vi "Main Tclk.vi"() -> ()   [LabVIEW 2018] (continued)
            n5536 = call "2D array edit.vi"("Auto close (s)"=u32 15, "Display Format:Precision"=u8 3, "Rows"=w5117, "Columns"=w5118, "Caption.Text"="Focus Index", "Input array"=w5115) -> ()  [unwired: 5 in, 1 out]
          }
          event "Pre-reheat Y stig": Mouse Down {
            n5537 = event-data() -> ()  [unwired: 9 out]
            n5538 = local read "Pre-reheat Y stig"() -> (w5122:sgl[][])
            n5539 = local read "SEM Scan Parameters"() -> (w5126:T26)
            n5540 = Unbundle By Name(w5126) -> ("X tiles"=w5125:u8, "Y tiles"=w5124:u8)
            n5541 = call "2D array edit.vi"("Auto close (s)"=u32 15, "Display Format:Precision"=u8 2, "Rows"=w5124, "Columns"=w5125, "Caption.Text"="Pre-reheat Y stig (%)", "Input array"=w5122) -> ()  [unwired: 5 in, 1 out]
          }
          event "Align failed array": Mouse Down {
            n5542 = event-data() -> ()  [unwired: 9 out]
            n5543 = local read "Align failed array"() -> (w5129:bool[][])
            n5544 = call "2D boolean array show.vi"("Input array"=w5129, "Caption.Text"="Align failed", "Colors [4]"=cluster{u32, u32}[] [{5898240, 5898240}, {16711680, 16711680}, {1985280, 1985280}, {6618880, 6618880}] ("Colors [4] 3")) -> ()  [unwired: 8 in]
          }
          event "AF Success tiled": Mouse Down {
            n5545 = event-data() -> ()  [unwired: 9 out]
            n5546 = local read "AF Success tiled"() -> (w5132:bool[][])
            n5547 = call "2D boolean array show.vi"("Input array"=w5132, "Caption.Text"="Auto Focus Success", "Colors [4]"=cluster{u32, u32}[] [{1985280, 1985280}, {6618880, 6618880}, {1985280, 1985280}, {6618880, 6618880}]) -> ()  [unwired: 8 in]
          }
          event "ASX Success tiled": Mouse Down {
            n5548 = event-data() -> ()  [unwired: 9 out]
            n5549 = local read "ASX Success tiled"() -> (w5135:bool[][])
            n5550 = call "2D boolean array show.vi"("Input array"=w5135, "Caption.Text"="Auto Stig X Success", "Colors [4]"=cluster{u32, u32}[] [{1985280, 1985280}, {6618880, 6618880}, {1985280, 1985280}, {6618880, 6618880}]) -> ()  [unwired: 8 in]
          }
          event "ASY Success tiled": Mouse Down {
            n5551 = event-data() -> ()  [unwired: 9 out]
            n5552 = local read "ASY Success tiled"() -> (w5138:bool[][])
            n5553 = call "2D boolean array show.vi"("Input array"=w5138, "Caption.Text"="Auto Stig Y Success", "Colors [4]"=cluster{u32, u32}[] [{1985280, 1985280}, {6618880, 6618880}, {1985280, 1985280}, {6618880, 6618880}]) -> ()  [unwired: 8 in]
          }
          event "AAX Success tiled": Mouse Down {
            n5554 = event-data() -> ()  [unwired: 9 out]
            n5555 = local read "AAX Success tiled"() -> (w5141:bool[][])
            n5556 = call "2D boolean array show.vi"("Input array"=w5141, "Caption.Text"="Auto Align X Success", "Colors [4]"=cluster{u32, u32}[] [{1985280, 1985280}, {6618880, 6618880}, {1985280, 1985280}, {6618880, 6618880}]) -> ()  [unwired: 8 in]
          }
          event "AAY Success tiled": Mouse Down {
            n5557 = event-data() -> ()  [unwired: 9 out]
            n5558 = local read "AAY Success tiled"() -> (w5144:bool[][])
            n5559 = call "2D boolean array show.vi"("Input array"=w5144, "Caption.Text"="Auto Align Y Success", "Colors [4]"=cluster{u32, u32}[] [{1985280, 1985280}, {6618880, 6618880}, {1985280, 1985280}, {6618880, 6618880}]) -> ()  [unwired: 8 in]
          }
          event "Best WD (mm) tiled": Mouse Down {
            n5560 = event-data() -> ()  [unwired: 9 out]
            n5561 = local read "Best WD (mm) tiled"() -> (w5147:dbl[][])
            n5562 = local read "SEM Scan Parameters"() -> (w5151:T26)
            n5563 = Unbundle By Name(w5151) -> ("X tiles"=w5150:u8, "Y tiles"=w5149:u8)
            n5564 = call "2D array edit.vi"("Auto close (s)"=u32 15, "Display Format:Precision"=u8 4, "Rows"=w5149, "Columns"=w5150, "Caption.Text"="Best WD (mm)", "Input array"=w5147) -> ()  [unwired: 5 in, 1 out]
          }
          event "Best Stig X (%) tiled": Mouse Down {
            n5565 = event-data() -> ()  [unwired: 9 out]
            n5566 = local read "Best Stig X (%) tiled"() -> (w5154:dbl[][])
            n5567 = local read "SEM Scan Parameters"() -> (w5158:T26)
            n5568 = Unbundle By Name(w5158) -> ("X tiles"=w5157:u8, "Y tiles"=w5156:u8)
            n5569 = call "2D array edit.vi"("Auto close (s)"=u32 15, "Display Format:Precision"=u8 2, "Rows"=w5156, "Columns"=w5157, "Caption.Text"="Best Stig X (%)", "Input array"=w5154) -> ()  [unwired: 5 in, 1 out]
          }
          event "Best Stig Y (%) tiled": Mouse Down {
            n5570 = event-data() -> ()  [unwired: 9 out]
            n5571 = local read "Best Stig Y (%) tiled"() -> (w5161:dbl[][])
            n5572 = local read "SEM Scan Parameters"() -> (w5165:T26)
            n5573 = Unbundle By Name(w5165) -> ("X tiles"=w5164:u8, "Y tiles"=w5163:u8)
            n5574 = call "2D array edit.vi"("Auto close (s)"=u32 15, "Display Format:Precision"=u8 2, "Rows"=w5163, "Columns"=w5164, "Caption.Text"="Best Stig Y (%)", "Input array"=w5161) -> ()  [unwired: 5 in, 1 out]
          }
          event "Best Aln X (%) tiled": Mouse Down {
            n5575 = event-data() -> ()  [unwired: 9 out]
            n5576 = local read "Best Aln X (%) tiled"() -> (w5168:dbl[][])
            n5577 = local read "SEM Scan Parameters"() -> (w5172:T26)
            n5578 = Unbundle By Name(w5172) -> ("X tiles"=w5171:u8, "Y tiles"=w5170:u8)
            n5579 = call "2D array edit.vi"("Auto close (s)"=u32 15, "Display Format:Precision"=u8 2, "Rows"=w5170, "Columns"=w5171, "Caption.Text"="Best Align X (%)", "Input array"=w5168) -> ()  [unwired: 5 in, 1 out]
          }
          event "Best Aln Y (%) tiled": Mouse Down {
            n5580 = event-data() -> ()  [unwired: 9 out]
            n5581 = local read "Best Aln Y (%) tiled"() -> (w5175:dbl[][])
            n5582 = local read "SEM Scan Parameters"() -> (w5179:T26)
            n5583 = Unbundle By Name(w5179) -> ("X tiles"=w5178:u8, "Y tiles"=w5177:u8)
            n5584 = call "2D array edit.vi"("Auto close (s)"=u32 15, "Display Format:Precision"=u8 2, "Rows"=w5177, "Columns"=w5178, "Caption.Text"="Best Align Y (%)", "Input array"=w5175) -> ()  [unwired: 5 in, 1 out]
          }
          event "Auto Focus Graph": Mouse Down {
            n5585 = event-data() -> ("PlatMods"=w5191:T77)  [unwired: 8 out]
            n5586 = Unbundle By Name(w5191) -> ("Shift"=w5190:bool)
            n5587 = local read "AF Graph scales tiled"() -> (w5187:cluster{sgl, sgl, sgl, sgl}[][])
            n5588 = local read "Auto Focus Graph tiled"() -> (w5196:T4)
            n5589 = local read "AF Y tile"() -> (w5195:u8)
            n5590 = local read "AF X tile"() -> (w5194:u8)
            n5591 = local read "SEM Scan Parameters"() -> (w5193:T26)
            n5592 = Unbundle By Name(w5193) -> ("X tiles"=w5192:u8, "Y tiles"=w5189:u8)
            n5593 = case shown="True" w5190 {
              tunnel: w5196 -> [w5206 w5215]
              tunnel: w5195 -> [w5199 w5213]
              tunnel: w5194 -> [w5205 w5208]
              tunnel: w5192 -> [w5203 _]
              tunnel: w5189 -> [_ w5214]
              tunnel: [w5202 w5212] -> w5188
              tunnel: w5187 -> [w5201 w5211]
              tunnel: [w5200 w5210] -> w5186
              tunnel: [w5197 w5207] -> w5181
              frame False {
                n5594 = Increment(x=w5205) -> (x+1=w5204:u8)
                n5595 = Quotient & Remainder(x=w5204, y=w5203) -> (x-y*floor(x/y)=w5198:u8)  [unwired: 1 out]
                n5596 = Index Array(array=w5201, index (row)=w5199, index (col)=w5198) -> (element=w5200:cluster{sgl, sgl, sgl, sgl})
                n5597 = Index Array(array=w5206, index (dim 0)=w5199, index (dim 1)=w5198) -> (element=w5202:T76)  [unwired: 1 in]
                n5598 = local write "AF X tile"(w5198) -> ()
                n5599 = Build Array(w5199, w5198) -> (w5197:u8[])
              }
              frame True {
                n5600 = Increment(x=w5213) -> (x+1=w5216:u8)
                n5601 = Quotient & Remainder(x=w5216, y=w5214) -> (x-y*floor(x/y)=w5209:u8)  [unwired: 1 out]
                n5602 = Index Array(array=w5211, index (row)=w5209, index (col)=w5208) -> (element=w5210:cluster{sgl, sgl, sgl, sgl})
                n5603 = Index Array(array=w5215, index (dim 0)=w5209, index (dim 1)=w5208) -> (element=w5212:T76)  [unwired: 1 in]
                n5604 = local write "AF Y tile"(w5209) -> ()
                n5605 = Build Array(w5209, w5208) -> (w5207:u8[])
              }
            }
            n5606 = Unbundle(w5186) -> (w5185:sgl, w5184:sgl, w5183:sgl, w5182:sgl)
            n5607 = local write "Auto Focus Graph"(w5188) -> ()
            n5608 = property on="AF Success tiled" class="Arr (strict)"("Index Values"=w5181) -> ()  [unwired: 2 in, 2 out]
            n5609 = property on="Best WD (mm) tiled" class="Arr (strict)"("Index Values"=w5181) -> ()  [unwired: 2 in, 2 out]
            n5610 = property on="Best WD FI tiled" class="Arr (strict)"("Index Values"=w5181) -> ()  [unwired: 2 in, 2 out]
            n5611 = property on="Auto Focus Graph" class="XYGraph (strict)"("XScale.Maximum"=w5185, "XScale.Minimum"=w5184, "YScale.Maximum"=w5183, "YScale.Minimum"=w5182) -> ()  [unwired: 2 in, 2 out]
          }
          event "Auto Stig X": Mouse Down {
            n5612 = event-data() -> ("PlatMods"=w5227:T77)  [unwired: 8 out]
            n5613 = Unbundle By Name(w5227) -> ("Shift"=w5226:bool)
            n5614 = local read "ASX Graph scales tiled"() -> (w5223:cluster{sgl, sgl, sgl, sgl}[][])
            n5615 = local read "ASX Graph tiled"() -> (w5232:T4)
            n5616 = local read "ASX Y tile"() -> (w5231:u8)
            n5617 = local read "ASX X tile"() -> (w5230:u8)
            n5618 = local read "SEM Scan Parameters"() -> (w5229:T26)
            n5619 = Unbundle By Name(w5229) -> ("X tiles"=w5228:u8, "Y tiles"=w5225:u8)
            n5620 = case shown="False" w5226 {
              tunnel: w5232 -> [w5242 w5251]
              tunnel: w5231 -> [w5235 w5249]
              tunnel: w5230 -> [w5241 w5244]
              tunnel: w5228 -> [w5239 _]
              tunnel: w5225 -> [_ w5250]
              tunnel: [w5238 w5248] -> w5224
              tunnel: w5223 -> [w5237 w5247]
              tunnel: [w5236 w5246] -> w5222
              tunnel: [w5233 w5243] -> w5217
              frame False {
                n5621 = Increment(x=w5241) -> (x+1=w5240:u8)
                n5622 = Quotient & Remainder(x=w5240, y=w5239) -> (x-y*floor(x/y)=w5234:u8)  [unwired: 1 out]
                n5623 = Index Array(array=w5237, index (row)=w5235, index (col)=w5234) -> (element=w5236:cluster{sgl, sgl, sgl, sgl})
                n5624 = Index Array(array=w5242, index (dim 0)=w5235, index (dim 1)=w5234) -> (element=w5238:T76)  [unwired: 1 in]
                n5625 = local write "ASX X tile"(w5234) -> ()
                n5626 = Build Array(w5235, w5234) -> (w5233:u8[])
              }
              frame True {
                n5627 = Increment(x=w5249) -> (x+1=w5252:u8)
                n5628 = Quotient & Remainder(x=w5252, y=w5250) -> (x-y*floor(x/y)=w5245:u8)  [unwired: 1 out]
                n5629 = Index Array(array=w5247, index (row)=w5245, index (col)=w5244) -> (element=w5246:cluster{sgl, sgl, sgl, sgl})
                n5630 = Index Array(array=w5251, index (dim 0)=w5245, index (dim 1)=w5244) -> (element=w5248:T76)  [unwired: 1 in]
                n5631 = local write "ASX Y tile"(w5245) -> ()
                n5632 = Build Array(w5245, w5244) -> (w5243:u8[])
              }
            }
            n5633 = Unbundle(w5222) -> (w5221:sgl, w5220:sgl, w5219:sgl, w5218:sgl)
            n5634 = local write "Auto Stig X"(w5224) -> ()
            n5635 = property on="ASX Success tiled" class="Arr (strict)"("Index Values"=w5217) -> ()  [unwired: 2 in, 2 out]
            n5636 = property on="Best Stig X (%) tiled" class="Arr (strict)"("Index Values"=w5217) -> ()  [unwired: 2 in, 2 out]
            n5637 = property on="Best Stig X FI tiled" class="Arr (strict)"("Index Values"=w5217) -> ()  [unwired: 2 in, 2 out]
            n5638 = property on="Auto Stig X" class="XYGraph (strict)"("XScale.Maximum"=w5221, "XScale.Minimum"=w5220, "YScale.Maximum"=w5219, "YScale.Minimum"=w5218) -> ()  [unwired: 2 in, 2 out]
          }
          event "Auto Stig Y": Mouse Down {
            n5639 = event-data() -> ("PlatMods"=w5263:T77)  [unwired: 8 out]
            n5640 = Unbundle By Name(w5263) -> ("Shift"=w5262:bool)
            n5641 = local read "ASY Graph scales tiled"() -> (w5259:cluster{sgl, sgl, sgl, sgl}[][])
            n5642 = local read "ASY Graph tiled"() -> (w5268:T4)
            n5643 = local read "ASY Y tile"() -> (w5267:u8)
            n5644 = local read "ASY X tile"() -> (w5266:u8)
            n5645 = local read "SEM Scan Parameters"() -> (w5265:T26)
            n5646 = Unbundle By Name(w5265) -> ("X tiles"=w5264:u8, "Y tiles"=w5261:u8)
            n5647 = case shown="True" w5262 {
              tunnel: w5268 -> [w5278 w5287]
              tunnel: w5267 -> [w5271 w5285]
              tunnel: w5266 -> [w5277 w5280]
              tunnel: w5264 -> [w5275 _]
              tunnel: w5261 -> [_ w5286]
              tunnel: [w5274 w5284] -> w5260
              tunnel: w5259 -> [w5273 w5283]
              tunnel: [w5272 w5282] -> w5258
              tunnel: [w5269 w5279] -> w5253
              frame False {
                n5648 = Increment(x=w5277) -> (x+1=w5276:u8)
                n5649 = Quotient & Remainder(x=w5276, y=w5275) -> (x-y*floor(x/y)=w5270:u8)  [unwired: 1 out]
                n5650 = Index Array(array=w5273, index (row)=w5271, index (col)=w5270) -> (element=w5272:cluster{sgl, sgl, sgl, sgl})
                n5651 = Index Array(array=w5278, index (dim 0)=w5271, index (dim 1)=w5270) -> (element=w5274:T76)  [unwired: 1 in]
                n5652 = local write "ASY X tile"(w5270) -> ()
                n5653 = Build Array(w5271, w5270) -> (w5269:u8[])
              }
              frame True {
                n5654 = Increment(x=w5285) -> (x+1=w5288:u8)
                n5655 = Quotient & Remainder(x=w5288, y=w5286) -> (x-y*floor(x/y)=w5281:u8)  [unwired: 1 out]
                n5656 = Index Array(array=w5283, index (row)=w5281, index (col)=w5280) -> (element=w5282:cluster{sgl, sgl, sgl, sgl})
                n5657 = Index Array(array=w5287, index (dim 0)=w5281, index (dim 1)=w5280) -> (element=w5284:T76)  [unwired: 1 in]
                n5658 = local write "ASY Y tile"(w5281) -> ()
                n5659 = Build Array(w5281, w5280) -> (w5279:u8[])
              }
            }
            n5660 = Unbundle(w5258) -> (w5257:sgl, w5256:sgl, w5255:sgl, w5254:sgl)
            n5661 = local write "Auto Stig Y"(w5260) -> ()
            n5662 = property on="ASY Success tiled" class="Arr (strict)"("Index Values"=w5253) -> ()  [unwired: 2 in, 2 out]
            n5663 = property on="Best Stig Y (%) tiled" class="Arr (strict)"("Index Values"=w5253) -> ()  [unwired: 2 in, 2 out]
            n5664 = property on="Best Stig Y FI tiled" class="Arr (strict)"("Index Values"=w5253) -> ()  [unwired: 2 in, 2 out]
            n5665 = property on="Auto Stig Y" class="XYGraph (strict)"("XScale.Maximum"=w5257, "XScale.Minimum"=w5256, "YScale.Maximum"=w5255, "YScale.Minimum"=w5254) -> ()  [unwired: 2 in, 2 out]
          }
          event "Auto Aln X": Mouse Down {
            n5666 = event-data() -> ("PlatMods"=w5299:T77)  [unwired: 8 out]
            n5667 = Unbundle By Name(w5299) -> ("Shift"=w5298:bool)
            n5668 = local read "AAX Graph scales tiled"() -> (w5295:cluster{sgl, sgl, sgl, sgl}[][])
            n5669 = local read "AAX Graph tiled"() -> (w5304:T4)
            n5670 = local read "AAX Y tile"() -> (w5303:u8)
            n5671 = local read "AAX X tile"() -> (w5302:u8)
            n5672 = local read "SEM Scan Parameters"() -> (w5301:T26)
            n5673 = Unbundle By Name(w5301) -> ("X tiles"=w5300:u8, "Y tiles"=w5297:u8)
            n5674 = case shown="False" w5298 {
              tunnel: w5304 -> [w5314 w5323]
              tunnel: w5303 -> [w5307 w5321]
              tunnel: w5302 -> [w5313 w5316]
              tunnel: w5300 -> [w5311 _]
              tunnel: w5297 -> [_ w5322]
              tunnel: [w5310 w5320] -> w5296
              tunnel: w5295 -> [w5309 w5319]
              tunnel: [w5308 w5318] -> w5294
              tunnel: [w5305 w5315] -> w5289
              frame False {
                n5675 = Increment(x=w5313) -> (x+1=w5312:u8)
                n5676 = Quotient & Remainder(x=w5312, y=w5311) -> (x-y*floor(x/y)=w5306:u8)  [unwired: 1 out]
                n5677 = local write "AAX X tile"(w5306) -> ()
                n5678 = Index Array(array=w5309, index (row)=w5307, index (col)=w5306) -> (element=w5308:cluster{sgl, sgl, sgl, sgl})
                n5679 = Index Array(array=w5314, index (dim 0)=w5307, index (dim 1)=w5306) -> (element=w5310:T76)  [unwired: 1 in]
                n5680 = Build Array(w5307, w5306) -> (w5305:u8[])
              }
              frame True {
                n5681 = Increment(x=w5321) -> (x+1=w5324:u8)
                n5682 = Quotient & Remainder(x=w5324, y=w5322) -> (x-y*floor(x/y)=w5317:u8)  [unwired: 1 out]
                n5683 = local write "AAX Y tile"(w5317) -> ()
                n5684 = Index Array(array=w5319, index (row)=w5317, index (col)=w5316) -> (element=w5318:cluster{sgl, sgl, sgl, sgl})
                n5685 = Index Array(array=w5323, index (dim 0)=w5317, index (dim 1)=w5316) -> (element=w5320:T76)  [unwired: 1 in]
                n5686 = Build Array(w5317, w5316) -> (w5315:u8[])
              }
            }
            n5687 = Unbundle(w5294) -> (w5293:sgl, w5292:sgl, w5291:sgl, w5290:sgl)
            n5688 = property on="AAX Success tiled" class="Arr (strict)"("Index Values"=w5289) -> ()  [unwired: 2 in, 2 out]
            n5689 = property on="Best Aln X (%) tiled" class="Arr (strict)"("Index Values"=w5289) -> ()  [unwired: 2 in, 2 out]
            n5690 = property on="Best Aln X FI tiled" class="Arr (strict)"("Index Values"=w5289) -> ()  [unwired: 2 in, 2 out]
            n5691 = local write "Auto Aln X"(w5296) -> ()
            n5692 = property on="Auto Aln X" class="XYGraph (strict)"("XScale.Maximum"=w5293, "XScale.Minimum"=w5292, "YScale.Maximum"=w5291, "YScale.Minimum"=w5290) -> ()  [unwired: 2 in, 2 out]
          }
          event "Auto Aln Y": Mouse Down {
            n5693 = event-data() -> ("PlatMods"=w5335:T77)  [unwired: 8 out]
            n5694 = Unbundle By Name(w5335) -> ("Shift"=w5334:bool)
            n5695 = local read "AAY Graph scales tiled"() -> (w5331:cluster{sgl, sgl, sgl, sgl}[][])
            n5696 = local read "AAY Graph tiled"() -> (w5340:T4)
            n5697 = local read "AAY Y tile"() -> (w5339:u8)
            n5698 = local read "AAY X tile"() -> (w5338:u8)
            n5699 = local read "SEM Scan Parameters"() -> (w5337:T26)
            n5700 = Unbundle By Name(w5337) -> ("X tiles"=w5336:u8, "Y tiles"=w5333:u8)
            n5701 = case shown="True" w5334 {
              tunnel: w5340 -> [w5350 w5359]
              tunnel: w5339 -> [w5343 w5357]
              tunnel: w5338 -> [w5349 w5352]
              tunnel: w5336 -> [w5347 _]
              tunnel: w5333 -> [_ w5358]
              tunnel: [w5346 w5356] -> w5332
              tunnel: w5331 -> [w5345 w5355]
              tunnel: [w5344 w5354] -> w5330
              tunnel: [w5341 w5351] -> w5325
              frame False {
                n5702 = Increment(x=w5349) -> (x+1=w5348:u8)
                n5703 = Quotient & Remainder(x=w5348, y=w5347) -> (x-y*floor(x/y)=w5342:u8)  [unwired: 1 out]
                n5704 = local write "AAY X tile"(w5342) -> ()
                n5705 = Index Array(array=w5345, index (row)=w5343, index (col)=w5342) -> (element=w5344:cluster{sgl, sgl, sgl, sgl})
                n5706 = Index Array(array=w5350, index (dim 0)=w5343, index (dim 1)=w5342) -> (element=w5346:T76)  [unwired: 1 in]
                n5707 = Build Array(w5343, w5342) -> (w5341:u8[])
              }
              frame True {
                n5708 = Increment(x=w5357) -> (x+1=w5360:u8)
                n5709 = Quotient & Remainder(x=w5360, y=w5358) -> (x-y*floor(x/y)=w5353:u8)  [unwired: 1 out]
                n5710 = local write "AAY Y tile"(w5353) -> ()
                n5711 = Index Array(array=w5355, index (row)=w5353, index (col)=w5352) -> (element=w5354:cluster{sgl, sgl, sgl, sgl})
                n5712 = Index Array(array=w5359, index (dim 0)=w5353, index (dim 1)=w5352) -> (element=w5356:T76)  [unwired: 1 in]
                n5713 = Build Array(w5353, w5352) -> (w5351:u8[])
              }
            }
            n5714 = Unbundle(w5330) -> (w5329:sgl, w5328:sgl, w5327:sgl, w5326:sgl)
            n5715 = property on="AAY Success tiled" class="Arr (strict)"("Index Values"=w5325) -> ()  [unwired: 2 in, 2 out]
            n5716 = property on="Best Aln Y (%) tiled" class="Arr (strict)"("Index Values"=w5325) -> ()  [unwired: 2 in, 2 out]
            n5717 = property on="Best Aln Y FI tiled" class="Arr (strict)"("Index Values"=w5325) -> ()  [unwired: 2 in, 2 out]
            n5718 = local write "Auto Aln Y"(w5332) -> ()
            n5719 = property on="Auto Aln Y" class="XYGraph (strict)"("XScale.Maximum"=w5329, "XScale.Minimum"=w5328, "YScale.Maximum"=w5327, "YScale.Minimum"=w5326) -> ()  [unwired: 2 in, 2 out]
          }
        }
        n5720 = Unbundle By Name(w2953) -> ("status"=w2951:bool)
        n5721 = Or(x=w2951, y=w2950) -> (x .or. y?=w2952:bool)
      }
      n5722 = while {
        stop <- w768 stop-if-true
        n5723 = Wait Until Next ms Multiple(millisecond multiple=u32 100) -> ()  [unwired: 1 out]
        n5724 = case shown="True" "Start Reheat" {
          frame False {
          }
          frame True {
            n5725 = stacked-sequence {
              frame #0 {
                n5726 = local read "Milling para"() -> (w773:T35)
                n5727 = local read "Auto reheat running"() -> (w771:bool)
                n5728 = Unbundle By Name(w773) -> ("Auto Profile"=w772:bool)
                n5729 = And(x=w772, y=w771) -> (x .and. y?=w770:bool)
                n5730 = case shown="True" w770 {
                  frame False {
                  }
                  frame True {
                    n5731 = stacked-sequence {
                      frame #0 {
                        n5732 = local read "Post #1up"() -> (w778:tag)
                        n5733 = local read "Post #1down"() -> (w777:tag)
                        n5734 = local read "Post #2up"() -> (w776:tag)
                        n5735 = local read "Post #2down"() -> (w775:tag)
                        n5736 = local write "FIB Profile"(TRUE ("FIB Profile")) -> ()
                        n5737 = local write "Enable logging"(FALSE ("Enable logging")) -> ()
                        n5738 = call "SEM shutter.vi"("Shutter close"=TRUE, "Shutter AO4"=w775, "Shutter AO3"=w776, "Shutter AO2"=w777, "Shutter AO1"=w778) -> ()  [unwired: 6 in, 1 out]
                      }
                      frame #1 {
                        n5739 = Wait (ms)(milliseconds to wait=u32 10000) -> ()  [unwired: 1 out]
                      }
                      frame #2 {
                        n5740 = local read "Machine Type"() -> (w782:u8)
                        n5741 = case shown="0, Default" w782 {
                          frame 0, Default {
                            w783 = sgl 90.0 ("UL-Ang")
                            n5742 = local read "HV Data Output"() -> (w799:T18)
                            n5743 = local read "Active logging channels"() -> (w787:string)
                            n5744 = local read "FIB HW Config"() -> (w790:T23)
                            n5745 = local read "FIB Options"() -> (w789:T33)
                            n5746 = local read "Milling para"() -> (w793:T35)
                            n5747 = local read "FIB profile X center (um)"() -> (w798:dbl)
                            n5748 = local read "FIB profile Y center (um)"() -> (w797:dbl)
                            n5749 = local read "FIB Scan Parameters"() -> (w792:T32)
                            n5750 = local read "Parameter Names"() -> (w786:string[])
                            n5751 = Bundle By Name(cluster=w792, "Frame line rampdown ratio"=0.0, "Oversampling"=u16 5) -> (w788:T32)
                            n5752 = Bundle By Name(cluster=w793, "X size (um)"=sgl 0.1, "Z size (um)"=sgl 10.0 ("Y size (um)"), "X center (um)"=w798, "Z center (um)"=w797, "UL-Ang"=w783, "UR-Ang"=w783) -> (w794:T35)
                            n5753 = call "FIB profile.vi"("HV Data Output"=w799, "Parameter Names"=w786, "Active logging channels"=w787, "Scan Para"=w788, "Milling para"=w794, "Options"=w789, "HW Config"=w790) -> ("Measurements"=w785:dbl[][])  [unwired: 2 in, 2 out]
                            n5754 = local write "Measurements"(w785) -> ()
                          }
                          frame 2 {
                            w800 = sgl 90.0 ("UL-Ang")
                            n5755 = local read "Active logging channels"() -> (w805:string)
                            n5756 = local read "FIB HW Config"() -> (w808:T23)
                            n5757 = local read "FIB Options"() -> (w807:T33)
                            n5758 = local read "Milling para"() -> (w811:T35)
                            n5759 = local read "FIB profile X center (um)"() -> (w816:dbl)
                            n5760 = local read "FIB profile Y center (um)"() -> (w815:dbl)
                            n5761 = local read "FIB Scan Parameters"() -> (w810:T32)
                            n5762 = local read "Parameter Names"() -> (w804:string[])
                            n5763 = local read "Capella HV Data Output"() -> (w801:T17)
                            n5764 = Bundle By Name(cluster=w810, "Frame line rampdown ratio"=0.0, "Oversampling"=u16 5) -> (w806:T32)
                            n5765 = Bundle By Name(cluster=w811, "X size (um)"=sgl 0.1, "Z size (um)"=sgl 10.0 ("Y size (um)"), "X center (um)"=w816, "Z center (um)"=w815, "UL-Ang"=w800, "UR-Ang"=w800) -> (w812:T35)
                            n5766 = call "FIB profile.vi"("Capella HV Data Output"=w801, "Parameter Names"=w804, "Active logging channels"=w805, "Scan Para"=w806, "Milling para"=w812, "Options"=w807, "HW Config"=w808) -> ("Measurements"=w803:dbl[][])  [unwired: 2 in, 2 out]
                            n5767 = local write "Measurements"(w803) -> ()
                          }
                        }
                      }
                      frame #3 {
                        n5768 = local write "FIB Profile"(FALSE ("FIB Profile")) -> ()
                        n5769 = local write "Enable logging"(TRUE ("Enable logging")) -> ()
                      }
                    }
                  }
                }
              }
              frame #1 {
                n5770 = local read "Machine Type"() -> (w819:u8)
                n5771 = case shown="2" w819 {
                  selector: w819 -> [w820 _ w911]
                  frame 0, Default {
                    n5772 = stacked-sequence {
                      tunnel: w820 -> [_ _ _ _ _ _ _ _ w905]
                      frame #0 {
                        n5773 = local read "Reheat start file"() -> (w821:path)
                        n5774 = File/Directory Info(path=w821) -> (path out=w824:path, error out=w822:errorcluster)  [unwired: 1 in, 5 out]
                        n5775 = Unbundle By Name(w822) -> ("status"=w823:bool)
                        n5776 = case shown="False" w823 {
                          tunnel: w824 -> [w825 _]
                          frame False {
                            n5777 = Delete(path (use dialog)=w825) -> ()  [unwired: 4 in, 3 out]
                          }
                          frame True {
                          }
                        }
                      }
                      frame #1 {
                        n5778 = local read "Reheat complete file"() -> (w828:path)
                        n5779 = local read "Reheat stopped file"() -> (w827:path)
                        n5780 = local write "Reheat completed"(FALSE ("Reheat completed")) -> ()
                        n5781 = local write "Status Tabs"(T11."FIB" ("Status Tabs")) -> ()
                        n5782 = File/Directory Info(path=w828) -> (path out=w834:path, last mod=w830:timestamp, error out=w836:errorcluster)  [unwired: 1 in, 4 out]
                        n5783 = File/Directory Info(path=w827) -> (path out=w833:path, error out=w831:errorcluster)  [unwired: 1 in, 5 out]
                        n5784 = Unbundle By Name(w836) -> ("status"=w835:bool)
                        n5785 = Unbundle By Name(w831) -> ("status"=w832:bool)
                        n5786 = case shown="False" w835 {
                          tunnel: w834 -> [w839 _]
                          tunnel: w830 -> [w838 _]
                          frame False {
                            n5787 = Delete(path (use dialog)=w839) -> ()  [unwired: 4 in, 3 out]
                            "Last auto reheat" <- w838
                          }
                          frame True {
                          }
                        }
                        n5788 = case shown="False" w832 {
                          tunnel: w833 -> [w837 _]
                          frame False {
                            n5789 = Delete(path (use dialog)=w837) -> ()  [unwired: 4 in, 3 out]
                          }
                          frame True {
                          }
                        }
                      }
                      frame #2 {
                        n5790 = local read "Auto reheat running"() -> (w847:bool)
                        n5791 = Get Date/Time In Seconds() -> (seconds since 1Jan1904=w844:timestamp)
                        "Reheat time" <- w844
                        n5792 = local read "Last auto reheat"() -> (w843:timestamp)
                        n5793 = local read "Turn FIB Gun on"() -> (w840:bool)
                        n5794 = property on="Request to stop reheat" class="Bool (strict)"("DisabledEnum"=T44."Enabled" ("Disabled")) -> ()  [unwired: 2 in, 2 out]
                        n5795 = Subtract(x=w844, y=w843) -> (x-y=w851:dbl)
                        n5796 = expression code="x/60"(w851) -> (w850:dbl)
                        n5797 = Less Or Equal?(x=w850, y=120.0) -> (x <= y?=w848:bool)
                        n5798 = And(x=w847, y=w848) -> (x .and. y?=w842:bool)
                        n5799 = Or(x=w842, y=w840) -> (x .or. y?=w841:bool)
                        n5800 = case shown="True" w841 {
                          tunnel: "Reheat Parameters" -> [w853 w859]
                          tunnel: [w853 w855] -> w845
                          frame False {
                          }
                          frame True {
                            n5801 = Bundle By Name(cluster=w859, "Filament I (A)"=sgl 0.1, "Reheat time (s)"=sgl 1.0, "Calculate V/I slope"=FALSE, "Disable Reheat Retries"=TRUE) -> (w855:T1)
                          }
                        }
                        "Actual Reheat Parameters" <- w845
                      }
                      frame #3 {
                        n5802 = local read "Actual Reheat Parameters"() -> (w861:T1)
                        n5803 = call "Write FIB reheat file.vi"("Reheat Parameters"=w861) -> ()  [unwired: 11 in]
                        "Send reheat start email" <- TRUE
                      }
                      frame #4 {
                        n5804 = while {
                          stop <- w877 stop-if-true
                          n5805 = local read "Reheat complete file"() -> (w873:path)
                          n5806 = local read "Reheat stopped file"() -> (w874:path)
                          n5807 = Wait Until Next ms Multiple(millisecond multiple=u32 100) -> ()  [unwired: 1 out]
                          n5808 = File/Directory Info(path=w873) -> (path out=w869:path, error out=w868:errorcluster)  [unwired: 1 in, 5 out]
                          n5809 = File/Directory Info(path=w874) -> (path out=w870:path, error out=w871:errorcluster)  [unwired: 1 in, 5 out]
                          n5810 = local read "Stop"() -> (w878:bool)
                          n5811 = Unbundle By Name(w868) -> ("status"=w867:bool)
                          n5812 = Unbundle By Name(w871) -> ("status"=w872:bool)
                          n5813 = Not(x=w867) -> (.not. x?=w875:bool)
                          n5814 = Not(x=w872) -> (.not. x?=w876:bool)
                          n5815 = case shown="True" w875 {
                            selector: w875 -> [w885 w886]
                            tunnel: w869 -> [_ w887]
                            tunnel: [w885 w886] -> w864
                            frame False {
                            }
                            frame True {
                              "Reheat log file" <- w887
                            }
                          }
                          n5816 = case shown="True" w876 {
                            selector: w876 -> [w882 w883]
                            tunnel: w870 -> [_ w884]
                            tunnel: [w882 w883] -> w863
                            frame False {
                            }
                            frame True {
                              n5817 = local write "Reheat log file"(w884) -> ()
                            }
                          }
                          n5818 = Or(x=w864, y=w863) -> (x .or. y?=w866:bool)
                          n5819 = Or(x=w866, y=w878) -> (x .or. y?=w877:bool)
                          n5820 = case shown="True" "Stop Reheat" {
                            frame False {
                              n5821 = local write "Status message"("FIB reheat in progress..." ("Status message")) -> ()
                            }
                            frame True {
                              n5822 = local write "Status message"("Stopping FIB reheat" ("Status message")) -> ()
                              n5823 = call "Write FIB reheat file.vi"("Start"=FALSE) -> ()  [unwired: 11 in]
                            }
                          }
                        }
                      }
                      frame #5 {
                        n5824 = Wait (ms)(milliseconds to wait=u32 500) -> ()  [unwired: 1 out]
                      }
                      frame #6 {
                        w895 = u8 1 items=["HV Data", "Reheat"] ("Log file type")
                        n5825 = local read "Reheat log file"() -> (w897:path)
                        n5826 = call "Read FIB Log Files.vi"("Log file type"=w895, "Log file path"=w897) -> ("Reheat Output"=→"Reheat Output":T21)  [unwired: 8 in, 1 out]
                        n5827 = call "Read FIB Log Files.vi"("Log file path"=path "C:/Program Files (x86)/FEI Company/BDS/LogHVData.log") -> ("HV Data Output"=w890:T113)  [unwired: 9 in, 1 out]
                        n5828 = File/Directory Info(path=path "C:/Program Files (x86)/FEI Company/BDS/Reheat/Stop.txt" ("Log file path")) -> (path out=w894:path, error out=w892:errorcluster)  [unwired: 1 in, 5 out]
                        n5829 = local write "HV Data Output"(w890) -> ()
                        n5830 = Unbundle By Name(w892) -> ("status"=w893:bool)
                        n5831 = case shown="False" w893 {
                          tunnel: w894 -> [w898 _]
                          frame False {
                            n5832 = Delete(path (use dialog)=w898) -> ()  [unwired: 4 in, 3 out]
                          }
                          frame True {
                          }
                        }
                      }
                      frame #7 {
                        n5833 = local read "Stop Reheat"() -> (w901:bool)
                        n5834 = local read "Reheat Output"() -> (w900:T21)
                        n5835 = Unbundle By Name(w900) -> ("Reheat Success"=w899:bool)
                        n5836 = Select(t="Reheat Stopped" ("Status message"), s=w901, f="Reheat Completed" ("Status message")) -> (s? t:f=w904:string)
                        n5837 = local write "Status message"(w904) -> ()
                        n5838 = local write "Start FIB HV DataLog"(w899) -> ()
                      }
                      frame #8 {
                        n5839 = local read "Reheat Output"() -> (w908:T21)
                        n5840 = local read "FIB Reheat Log Files"() -> (w907:path)
                        n5841 = local read "Reheat time"() -> (w906:timestamp)
                        n5842 = local read "HV Data Output"() -> (w910:T18)
                        n5843 = local read "Actual Reheat Parameters"() -> (w909:T1)
                        n5844 = call "Write FIB reheat log.vi"("HV Data Output"=w910, "Reheat Output"=w908, "Reheat Parameters"=w909, "Reheat time"=w906, "Machine Type"=w905, "Log file path"=w907) -> ()  [unwired: 6 in]
                      }
                    }
                  }
                  frame 1 {
                  }
                  frame 2 {
                    n5845 = stacked-sequence {
                      tunnel: w911 -> [_ _ _ _ _ _ w1029]
                      frame #0 {
                        n5846 = local read "Api"() -> (w914:refnum<k7>)
                        n5847 = local write "Status Tabs"(T11."FIB" ("Status Tabs")) -> ()
                        n5848 = local write "Reheat completed"(FALSE ("Reheat completed")) -> ()
                        n5849 = property on="Request to stop reheat" class="Bool (strict)"("DisabledEnum"=T44."Enabled" ("Disabled")) -> ()  [unwired: 2 in, 2 out]
                        n5850 = call "SmartSEM Remote API set float.vi"("vValue"=sgl 1.0, "lpszParam"="DP_FIB_BLANKED", "Api"=w914) -> ("error out"=w912:errorcluster, "Api out"=w913:refnum<k7>)  [unwired: 7 in]
                        n5851 = call "SmartSEM Remote API get FIB HV data.vi"("error in"=w912, "Api in"=w913) -> ("Capella HV Data Output"=w917:T17)  [unwired: 6 in, 3 out]
                        n5852 = local write "Capella HV Data Output"(w917) -> ()
                      }
                      frame #1 {
                        n5853 = Get Date/Time In Seconds() -> (seconds since 1Jan1904=w921:timestamp)
                        n5854 = local read "Api"() -> (w924:refnum<k7>)
                        n5855 = local write "Send reheat start email"(TRUE) -> ()
                        n5856 = local write "Reheat time"(w921) -> ()
                        n5857 = invoke class="_EMApi" method="Execute"(reference=w924, "lpszCommand"="CMD_FIB_TC_MH_REQ_START") -> ()  [unwired: 2 in, 4 out]
                      }
                      frame #2 {
                        n5858 = Wait (ms)(milliseconds to wait=u32 30000) -> ()  [unwired: 1 out]
                        n5859 = local write "Status message"("FIB reheat in progress..." ("Status message")) -> ()
                      }
                      frame #3 {
                        n5860 = while {
                          stop <- w932 stop-if-true
                          n5861 = local read "Api"() -> (w929:refnum<k7>)
                          n5862 = call "SmartSEM Remote API FIB gun state.vi"("Api"=w929) -> ("FIB Gun State"=w931:string, "Api out"=w927:refnum<k7>)  [unwired: 8 in, 1 out]
                          n5863 = Wait Until Next ms Multiple(millisecond multiple=u32 100) -> ()  [unwired: 1 out]
                          n5864 = case shown="\"FIB Emissin Failed\"" w931 {
                            tunnel: [FALSE ("x") TRUE ("x") w949] -> w930
                            tunnel: w927 -> [_ _ w948]
                            frame "", Default {
                            }
                            frame "FIB Emissin Failed" {
                              n5865 = Get Date/Time In Seconds() -> (seconds since 1Jan1904=w938:timestamp)
                              n5866 = Get Date/Time String(seconds (now)=w938) -> (date string=w939:string, time string=w940:string)  [unwired: 2 in]
                              n5867 = Concatenate Strings(w939, " " ("string"), w940) -> (w937:string)
                              n5868 = local read "Reheat Output"() -> (w942:T21)
                              n5869 = Bundle By Name(cluster=w942, "Reheat finish time"=w937, "Reheat Success"=FALSE) -> (w943:T21)
                              n5870 = local write "Reheat Output"(w943) -> ()
                            }
                            frame "Regulating" {
                              n5871 = call "SmartSEM Remote API get string.vi"("lpszParam"="DP_FIB_PURGE_STATE", "Api"=w948) -> ("data"=w946:string, "Api out"=w945:refnum<k7>)  [unwired: 7 in, 1 out]
                              n5872 = case shown="\"Idle\"" w946 {
                                tunnel: w945 -> [_ w952]
                                tunnel: [FALSE ("x") w951] -> w949
                                frame "", Default {
                                }
                                frame "Idle" {
                                n5873 = stacked-sequence {
                                tunnel: w952 -> [w955 _ w960 _]
                                tunnel: [_ _ _ TRUE ("x")] -> w951
                                frame #0 {
                                n5874 = local read "FIB HW Config"() -> (w954:T23)
                                n5875 = Unbundle By Name(w954) -> ("Beam blank"=w953:tag)
                                n5876 = call "FIB beam blank.vi"("Api"=w955, "Beam blanked"=TRUE, "lines"=w953) -> ()  [unwired: 2 in, 1 out]
                                }
                                frame #1 {
                                n5877 = Wait (ms)(milliseconds to wait=u32 60000) -> ()  [unwired: 1 out]
                                n5878 = local write "Status message"("Stablizing for 1 min ..." ("Status message")) -> ()
                                }
                                frame #2 {
                                n5879 = call "SmartSEM Remote API FIB VI slope.vi"("Api"=w960) -> ("V/I slope"=w961:sgl)  [unwired: 8 in, 2 out]
                                n5880 = local write "Status message"("Measuring FIB V/I slope ..." ("Status message")) -> ()
                                n5881 = local write "FIB V/I slope"(w961) -> ()
                                }
                                frame #3 {
                                }
                                }
                                }
                              }
                            }
                          }
                          n5882 = local read "Stop Reheat"() -> (w928:bool)
                          n5883 = local read "Stop"() -> (w934:bool)
                          n5884 = Compound Arithmetic op=OR(w930, w934, w928) -> (w932:bool)
                        }
                      }
                      frame #4 {
                        n5885 = while {
                          stop <- w969 stop-if-true
                          n5886 = local read "Api"() -> (w965:refnum<k7>)
                          n5887 = call "SmartSEM Remote API FIB gun state.vi"("Api"=w965) -> ("FIB Gun State"=w968:string, "Api out"=w963:refnum<k7>)  [unwired: 8 in, 1 out]
                          n5888 = Wait Until Next ms Multiple(millisecond multiple=u32 100) -> ()  [unwired: 1 out]
                          n5889 = case shown="\"Regulating\"" w968 {
                            tunnel: [FALSE ("x") TRUE ("x") TRUE ("x") w991] -> w967
                            tunnel: w963 -> [_ _ _ w992]
                            frame "", Default {
                            }
                            frame "FIB Emissin Failed" {
                              n5890 = Get Date/Time In Seconds() -> (seconds since 1Jan1904=w975:timestamp)
                              n5891 = Get Date/Time String(seconds (now)=w975) -> (date string=w976:string, time string=w977:string)  [unwired: 2 in]
                              n5892 = Concatenate Strings(w976, " " ("string"), w977) -> (w974:string)
                              n5893 = local read "Reheat Output"() -> (w979:T21)
                              n5894 = Bundle By Name(cluster=w979, "Reheat finish time"=w974, "Reheat Success"=FALSE) -> (w980:T21)
                              n5895 = local write "Reheat Output"(w980) -> ()
                            }
                            frame "Standby" {
                              n5896 = Get Date/Time In Seconds() -> (seconds since 1Jan1904=w984:timestamp)
                              n5897 = Get Date/Time String(seconds (now)=w984) -> (date string=w985:string, time string=w986:string)  [unwired: 2 in]
                              n5898 = Concatenate Strings(w985, " " ("string"), w986) -> (w983:string)
                              n5899 = local read "Reheat Output"() -> (w988:T21)
                              n5900 = Bundle By Name(cluster=w988, "Reheat finish time"=w983, "Reheat Success"=FALSE) -> (w989:T21)
                              n5901 = local write "Reheat Output"(w989) -> ()
                            }
                            frame "Regulating" {
                              n5902 = stacked-sequence {
                                tunnel: w992 -> [w995 w1002]
                                tunnel: [_ w1003] -> w991
                                frame #0 {
                                n5903 = Wait (ms)(milliseconds to wait=u32 2000) -> ()  [unwired: 1 out]
                                n5904 = call "SmartSEM Remote API set float.vi"("vValue"=sgl 1.0, "lpszParam"="DP_FIB_BLANKED", "Api"=w995) -> ("error out"=w993:errorcluster, "Api out"=w994:refnum<k7>)  [unwired: 7 in]
                                n5905 = call "SmartSEM Remote API get FIB HV data.vi"("error in"=w993, "Api in"=w994) -> ("Capella HV Data Output"=w998:T17)  [unwired: 6 in, 3 out]
                                n5906 = local write "Capella HV Data Output"(w998) -> ()
                                }
                                frame #1 {
                                n5907 = call "SmartSEM Remote API get string.vi"("lpszParam"="DP_FIB_PURGE_STATE", "Api"=w1002) -> ("data"=w1000:string)  [unwired: 7 in, 2 out]
                                n5908 = case shown="\"Idle\"" w1000 {
                                tunnel: w1002 -> [_ w1006]
                                tunnel: [FALSE ("x") w1005] -> w1003
                                frame "", Default {
                                }
                                frame "Idle" {
                                n5909 = stacked-sequence {
                                tunnel: w1006 -> [_ w1017 _]
                                tunnel: [_ _ TRUE ("x")] -> w1005
                                frame #0 {
                                w1008 = TRUE ("Reheat Success")
                                n5910 = Get Date/Time In Seconds() -> (seconds since 1Jan1904=w1010:timestamp)
                                n5911 = local read "FIB V/I slope"() -> (w1007:sgl)
                                n5912 = Get Date/Time String(seconds (now)=w1010) -> (date string=w1011:string, time string=w1012:string)  [unwired: 2 in]
                                n5913 = Concatenate Strings(w1011, " " ("string"), w1012) -> (w1009:string)
                                n5914 = local read "Reheat Output"() -> (w1014:T21)
                                n5915 = Bundle By Name(cluster=w1014, "Reheat finish time"=w1009, "Reheat Success"=w1008, "V/I Slope"=w1007) -> (w1015:T21)
                                n5916 = local write "Start FIB HV DataLog"(w1008) -> ()
                                n5917 = local write "Reheat Output"(w1015) -> ()
                                }
                                frame #1 {
                                n5918 = call "SmartSEM Remote API FIB Gun Valve.vi"("FIB Gun Valve"=enum16{"Close", "Open"}."Open", "Api"=w1017) -> ()  [unwired: 8 in, 2 out]
                                }
                                frame #2 {
                                n5919 = local read "Reheat Output"() -> (w1022:T21)
                                n5920 = local read "Capella HV Data Output"() -> (w1020:T17)
                                n5921 = Unbundle By Name(w1020) -> ("Emission Actual (uA)"=w1019:sgl, "Suppressor (V)"=w1018:sgl)
                                n5922 = Bundle By Name(cluster=w1022, "Initial emission (uA)"=w1019, "Initial suppressor (V)"=w1018) -> (w1021:T21)
                                n5923 = local write "Reheat Output"(w1021) -> ()
                                }
                                }
                                }
